vi "String - Split Single Command and Access Control String.vi"(11 "Command and RW Property":string) -> (1 "Write Access":bool, 2 "Read Access":bool, 3 "Command":string)   [LabVIEW 2017, in "Communications Library.lvlib"]
doc: "Deciphers a single line from the response to the help2 command."
uses:
  Communications Library.lvlib
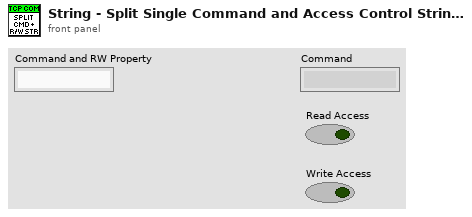
[diagram p1: front panel]
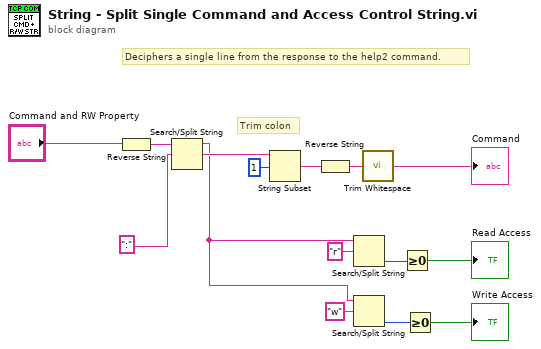
[diagram p0: block diagram]
diagram:
  # "Deciphers a single line from the response to the help2 command."
  # "Trim colon"
  n1 = Reverse String(1:"Command and RW Property") -> (0:w5:string)
  n2 = Search/Split String(string=w5, search string/char (-)=":") -> (substring before match=w1:string, match + rest of string=w3:string)  [unwired: 1 in, 1 out]
  n3 = String Subset(string=w3, offset (0)=1) -> (substring=w2:string)  [unwired: 1 in]
  n4 = Reverse String(1:w2) -> (0:w4:string)
  n5 = Search/Split String(string=w1, search string/char (-)="r") -> (offset of match=w12:i32)  [unwired: 1 in, 2 out]
  n6 = Search/Split String(string=w1, search string/char (-)="w") -> (offset of match=w13:i32)  [unwired: 1 in, 2 out]
  n7 = call <vilib>:"Trim Whitespace.vi"("string"=w4) -> ("trimmed string"=→"Command":string)  [unwired: 1 in]
  n8 = Greater Or Equal To 0?(x=w12) -> (x >= 0?=→"Read Access":bool)
  n9 = Greater Or Equal To 0?(x=w13) -> (x >= 0?=→"Write Access":bool)
